vi "Primary logic for trip prevention.vi"(7 "Barcodes in":string[](array[string]), 8 "VISA Refnum in":refnum<visa-resource-name>, 10 "Stop Program":bool) -> (0 "channel 3 currents":dbl[](array[numeric]), 1 "channel 4 currents":dbl[](array[numeric]), 3 "Power Supply Trip":bool, 4 "channel 2 currents":dbl[](array[numeric]), 6 "channel 1 currents":dbl[](array[numeric]))   [LabVIEW 2020]
uses:
  Program Files/National Instruments/LabVIEW 2018/instr.lib/CAEN PSM/CAEN PSM.lvlib
panel:
  out "BoardHandle out 2":T1
  out "error out":errorcluster
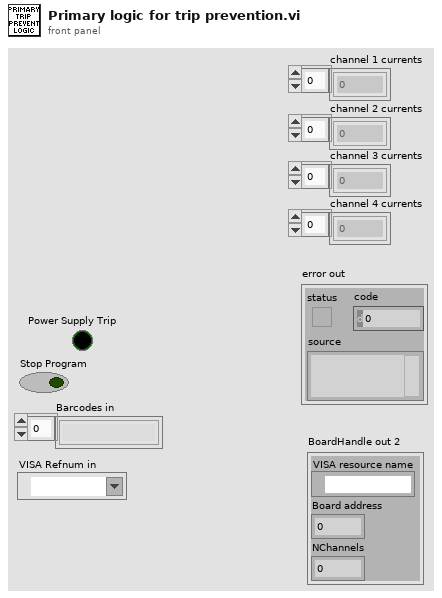
[diagram p1: front panel]
types:
  T1 = cluster{"VISA resource name":refnum<visa-resource-name>, "Board address":u8, "NChannels":u8}
  T2 = typedef "CAEN PSM.lvlib/BoardHandle.ctl" = cluster{"VISA resource name":refnum<visa-resource-name>, "Board address":u8, "NChannels":u8}
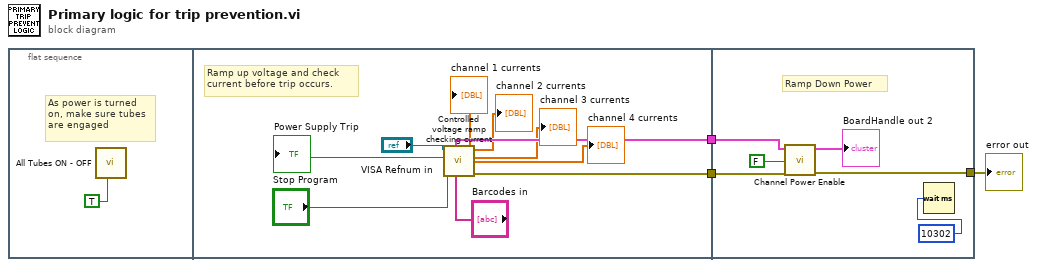
[diagram p0: block diagram]
diagram:
  n1 = flat-sequence {
    tunnel: [w13] -> w3
    tunnel: [w9] -> w1
    tunnel: w3 -> [w17]
    tunnel: [w16] -> w2
    tunnel: w1 -> [w15]
    frame #0 {
      # "As power is turned\non, make sure tubes\nare engaged"
      n2 = call "All Tubes ON - OFF.vi"("Tubes ON/OFF"=TRUE ("Activate: 1\nDeactivate: 0")) -> ()  [unwired: 11 in]
    }
    frame #1 {
      # "Ramp up voltage and check \ncurrent before trip occurs."
      n3 = call "Controlled voltage ramp checking current.vi"("Barcodes in"="Barcodes in", "Stop Program"="Stop Program", "VISA Refnum in"="VISA Refnum in") -> ("error out"=w13:errorcluster, "channel 4 currents"=→"channel 4 currents":dbl[], "channel 3 currents"=→"channel 3 currents":dbl[], "channel 2 currents"=→"channel 2 currents":dbl[], "channel 1 currents"=→"channel 1 currents":dbl[], "BoardHandle out 2"=w9:T1, "Power Supply Trip"=→"Power Supply Trip":bool)  [unwired: 2 in]
    }
    frame #2 {
      # "Ramp Down Power"
      n4 = call "Channel Power Enable.vi"("error in (no error)"=w17, "Enable (OFF)"=FALSE, "BoardHandle"=w15) -> ("error out"=w16:errorcluster, "BoardHandle out"=→"BoardHandle out 2":T2)  [unwired: 7 in]
      n5 = Wait (ms)(milliseconds to wait=u32 10302) -> ()  [unwired: 1 out]
    }
  }
  "error out" <- w2
